vi "Test Executive.vi"(11 "Module Config":T30={"Name"="Test Executive", "Parent Q"=refnum, "Is Child?"=FALSE, "Index"=0, "Dirs"={"Root"=path "C:/MTE", "Config"=path "C:/MTE/Config", "Logs"=path "C:/MTE/Logs", "Reports"=path "C:/ATE/Reports", "App Data"=path "C:/ProgramData/Test Executive"}, "Simulate"=FALSE, "SimCtrl"=refnum}) -> ()   [LabVIEW 2018] (continued)
            n1825 = Delete From Array(array=w3877, index=0) -> (deleted portion=w3874:string, array with subset deleted=w3876:string[])  [unwired: 1 in]
            n1826 = local read "StaCnct"() -> (w3871:bool)
            n1827 = case shown="True" w3871 {
              tunnel: w3876 -> [_ w3915]
              tunnel: w3875 -> [w3890 w3911]
              tunnel: w3874 -> [_ w3896]
              tunnel: w3873 -> [w3887 w3907]
              tunnel: [w3889 w3905] -> w3872
              tunnel: w3870 -> [_ w3898]
              frame False {
                n1828 = call "TestExec.Config, Get Station SW Module Info.vi"() -> ("Sta Exe Path"=w3882:path)  [unwired: 8 in, 3 out]
                n1829 = Strip Path(path=w3882) -> (name=w3881:string)  [unwired: 1 out]
                n1830 = Format Into String(format string="Cannot connect to the '%s'Test Station Applicaiton.\nMake sure it is correctly installed and is running." ("source"), w3881) -> (resulting string=w3883:string)  [unwired: 2 in, 1 out]
                n1831 = call <vilib>:"Q.Enqueue Seq.vi"("Seq Task Name"="Test Running", "Q In"=w3887) -> ()  [unwired: 8 in, 2 out]
                n1832 = Bundle By Name(cluster=errorcluster {"status"=TRUE, "code"=-5100, "source"=""} ("error constant"), "source"=w3883) -> (w3884:errorcluster)
                n1833 = Bundle By Name(cluster=w3890, "ResultError"=w3884) -> (w3889:T73)
              }
              frame True {
                # "Make timeout 10% longer."
                # "Send command to station"
                n1834 = Unbundle By Name(w3911) -> ("TimeOut(s)"=w3917:dbl, "StaApp"=w3912:string)
                n1835 = Multiply(x=1.1, y=w3917) -> (x*y=w3893:dbl)
                n1836 = To Variant(anything=w3915) -> (Variant=w3914:variant)
                n1837 = local read "Abort Flag"() -> (w3892:bool)
                n1838 = Max & Min(x=1.0, y=w3893) -> (min(x,y)=w3894:dbl)  [unwired: 1 out]
                n1839 = call <vilib>:"Q.Enqueue Function.vi"("RetSubCmd"="StaCmd_RTN", "Q Name"=w3912, "Data1"=w3914, "Task Name"=w3896, "Q In"=w3907) -> ("error out"=w3908:errorcluster, "SeqNum"=w3897:i32)  [unwired: 4 in, 1 out]
                n1840 = Select(t=w3894, s=w3892, f=w3893) -> (s? t:f=w3891:dbl)
                n1841 = To Variant(anything=w3896) -> (Variant=w3909:variant)
                n1842 = call <vilib>:"Scheduler.AddTask.vi"("Data1"=w3909, "Interval(s)"=w3891, "Error In"=w3908, "Task Name"="StaCmd_TIMEOUT", "Sched Name"=w3896, "Q In"=w3907) -> ("Error Out"=w3906:errorcluster)  [unwired: 4 in, 1 out]
                n1843 = Bundle By Name(cluster=w3911, "Funct.Seq"=w3897, "Funct.Name"=w3896, "ResultError"=w3906) -> (w3905:T73)
                n1844 = Format Into String(format string="Funct Init: Name \"%s\", Seq %d, TimeOut %#f.", w3896, w3897, w3891) -> (resulting string=w3904:string)  [unwired: 2 in, 1 out]
                n1845 = Unbundle By Name(w3898) -> ("Log"=w3903:refnum<class "Event Notification.lvclass">)
                n1846 = call <vilib>:"Event Notification.Status Message.vi"("Display"=FALSE, "Log"=TRUE, "Level"=Event_Log.Log_Level."Debug0", "Message"=w3904, "Event Notification in"=w3903) -> ()  [unwired: 7 in]
              }
            }
          }
          frame "StaCmd_RTN" {
            n1847 = local read "Abort Flag"() -> (w3919:bool)
            n1848 = Select(t="Done", s=w3919, f="Validate") -> (s? t:f=w3920:string)
            n1849 = while {
              shift-right: [w3935] -> w3924
              shift-left: w3928 -> [w3940]
              tunnel: w3927 -> [w3939]
              tunnel: w3926 -> [w3938]
              tunnel: w3925 -> [w3937]
              shift-right: [w3936] -> _
              shift-left: w3920 -> [w3929]
              tunnel: w3923 -> [w3933]
              shift-right: [w3932] -> _
              shift-left: _ -> [w3931]
              tunnel: w3922 -> [w3930]
              stop <- w3934 stop-if-true
              n1850 = case shown="\"Check Error\"" w3929 {
                tunnel: w3940 -> [w3955 w3964 w3967 w3985 w4007 w4013]
                tunnel: w3939 -> [_ _ w3970 _ _ _]
                tunnel: w3938 -> [w3961 _ _ _ _ _]
                tunnel: w3937 -> [_ _ _ _ _ _]
                tunnel: [w3956 "Load Vars" "Check Error" "Resume Seq" "Done" _] -> w3936
                tunnel: [w3955 w3964 w3971 w3988 w4006 w4013] -> w3935
                tunnel: [_ _ _ _ _ TRUE] -> w3934
                tunnel: w3933 -> [_ w3962 _ _ w4008 _]
                tunnel: [w3945 w3966 w3968 w3987 w4004 w4011] -> w3932
                tunnel: w3931 -> [_ w3966 w3968 w3987 w4004 w4011]
                tunnel: w3930 -> [w3949 _ _ _ _ _]
                frame "Validate" {
                  # "Ignore"
                  n1851 = Variant To Data(type=T55 {"SeqNum"=0, "Data"=variant, "Error"={"status"=FALSE, "code"=0, "source"=""}} ("Ret"), Variant=w3961) -> (data=w3945:T55)  [unwired: 1 in, 1 out]
                  n1852 = Unbundle By Name(w3955) -> ("Funct.Seq"=w3948:i32)
                  n1853 = Unbundle By Name(w3945) -> ("SeqNum"=w3960:i32)
                  n1854 = Unbundle By Name(w3945) -> ("Error.status"=w3944:bool)
                  n1855 = Equal?(x=w3948, y=w3960) -> (x = y?=w3959:bool)
                  n1856 = Select(t="Error", s=w3944, f="OK") -> (s? t:f=w3941:string)
                  n1857 = Select(t="Kill Timeout", s=w3959, f="Done") -> (s? t:f=w3956:string)
                  n1858 = Format Into String(format string="Funct RTN: Seq %d, Status %s", w3948, w3941) -> (resulting string=w3946:string)  [unwired: 2 in, 1 out]
                  n1859 = Unbundle By Name(w3949) -> ("Log"=w3953:refnum<class "Event Notification.lvclass">)
                  n1860 = call <vilib>:"Event Notification.Status Message.vi"("Display"=FALSE, "Log"=TRUE, "Level"=Event_Log.Log_Level."Debug0", "Message"=w3946, "Event Notification in"=w3953) -> ()  [unwired: 7 in]
                }
                frame "Kill Timeout" {
                  n1861 = Unbundle By Name(w3964) -> ("Funct.Name"=w3963:string)
                  n1862 = call <vilib>:"Scheduler.Delete Task.vi"("Sched Name"=w3963, "Q In"=w3962) -> ()  [unwired: 8 in, 2 out]
                }
                frame "Load Vars" {
                  n1863 = Variant To Data(type=string[][] [], Variant=w3970) -> (data=w3972:string[][], error out=w3973:errorcluster)  [unwired: 1 in]
                  n1864 = case shown="No Error" w3973 {
                    tunnel: w3972 -> [w3976 _]
                    tunnel: w3967 -> [w3981 w3982]
                    tunnel: [w3980 w3982] -> w3971
                    frame No Error {
                      n1865 = local read "Variables"() -> (w3977:string[][])
                      n1866 = Unbundle By Name(w3981) -> ("SeqMgr"=w3979:refnum<class "SeqMgr.lvclass">)
                      n1867 = call "TestExec.Add New 1D Items to 2D List, Overwrite if is existing.vi"("New Items"=w3976, "Item List"=w3977) -> ("Item List Out"=w3975:string[][])  [unwired: 9 in]
                      n1868 = call <vilib>:"SeqMgr.Variables - Add, Replace.vi"("Name, Value"=w3976, "SeqMgr in"=w3979) -> ("SeqMgr out"=w3978:refnum<class "SeqMgr.lvclass">)  [unwired: 8 in, 1 out]
                      n1869 = local write "Variables"(w3975) -> ()
                      n1870 = Bundle By Name(cluster=w3981, "SeqMgr"=w3978) -> (w3980:T73)
                    }
                    frame Error {
                      # "No data\nDo nothing"
                    }
                  }
                }
                frame "Check Error" {
                  n1871 = Unbundle By Name(w3985) -> ("Funct.Name"=w3984:string)
                  n1872 = Unbundle By Name(w3987) -> ("Error"=w3986:errorcluster)
                  n1873 = case shown="Error" w3986 {
                    selector: w3986 -> [_ w4001]
                    tunnel: w3984 -> [_ w3998]
                    tunnel: [_ w4000] -> w3983
                    frame No Error {
                    }
                    frame Error {
                      n1874 = Unbundle By Name(w4001) -> ("source"=w3991:string)
                      n1875 = Match Pattern(string=w3991, regular expression="Details = ") -> (after substring=w3992:string, offset past match=w3995:i32)  [unwired: 1 in, 2 out]
                      n1876 = Concatenate Strings("Action = ", w3998) -> (w3997:string)
                      n1877 = Greater Or Equal To 0?(x=w3995) -> (x >= 0?=w3993:bool)
                      n1878 = Select(t=w3992, s=w3993, f=w3991) -> (s? t:f=w3990:string)
                      n1879 = Concatenate Strings(w3997, ", Details = ", w3990) -> (w4002:string)
                      n1880 = Bundle By Name(cluster=w4001, "source"=w4002) -> (w4000:errorcluster)
                    }
                  }
                  n1881 = Bundle By Name(cluster=w3985, "ResultError"=w3983) -> (w3988:T73)
                }
                frame "Resume Seq" {
                  n1882 = call <vilib>:"Q.Enqueue Seq.vi"("Seq Task Name"="Test Running", "Q In"=w4008) -> ()  [unwired: 8 in, 2 out]
                  n1883 = Bundle By Name(cluster=w4007, "Funct.Seq"=0 ("FunctID"), "Funct.Name"="") -> (w4006:T73)
                }
                frame "Done", Default {
                }
              }
            }
          }
          frame "StaCmd_TIMEOUT" {
            n1884 = Unbundle By Name(w4021) -> ("Funct.Name"=w4014:string, "TimeOut(s)"=w4016:dbl, "Funct.Seq"=w4017:i32)
            n1885 = Empty String/Path?(string/path=w4014) -> (empty?=w4015:bool)
            n1886 = case shown="False" w4015 {
              tunnel: w4021 -> [w4041 w4046]
              tunnel: w4020 -> [w4036 _]
              tunnel: [w4032 w4046] -> w4019
              tunnel: w4018 -> [w4031 _]
              tunnel: w4014 -> [w4029 _]
              tunnel: w4017 -> [w4024 _]
              tunnel: w4016 -> [w4023 _]
              frame False {
                n1887 = local read "Test State"() -> (w4035:enum32{"Idle", "Running", "Completed"})
                n1888 = Equal?(x=w4035, y=enum32{"Idle", "Running", "Completed"}."Running" ("Test State")) -> (x = y?=w4033:bool)
                n1889 = case shown="True" w4033 {
                  tunnel: w4036 -> [_ w4044]
                  frame False {
                  }
                  frame True {
                    n1890 = call <vilib>:"Q.Enqueue Seq.vi"("Seq Task Name"="Test Running", "Q In"=w4044) -> ()  [unwired: 8 in, 2 out]
                  }
                }
                n1891 = Format Into String(format string="Function \"%s\" TIMED OUT.  There was no Response within %f# seconds.", w4029, w4023) -> (resulting string=w4038:string)  [unwired: 2 in, 1 out]
                n1892 = Bundle By Name(cluster=errorcluster {"status"=TRUE, "code"=-5100, "source"=""} ("error constant"), "source"=w4038) -> (w4037:errorcluster)
                n1893 = Bundle By Name(cluster=w4041, "Funct.Seq"=0, "Funct.Name"="", "ResultError"=w4037) -> (w4032:T73)
                n1894 = Format Into String(format string="Funct Timeout: Name \"%s\", Seq %d, Time %#f.", w4029, w4024, w4023) -> (resulting string=w4022:string)  [unwired: 2 in, 1 out]
                n1895 = Unbundle By Name(w4031) -> ("Log"=w4030:refnum<class "Event Notification.lvclass">)
                n1896 = call <vilib>:"Event Notification.Status Message.vi"("Display"=FALSE, "Log"=TRUE, "Level"=Event_Log.Log_Level."Verbose", "Message"=w4022, "Event Notification in"=w4030) -> ()  [unwired: 7 in]
              }
              frame True {
                # "Do nothing\nTime out was invalid"
              }
            }
          }
          frame "StaTest End" {
            n1897 = Unbundle By Name(w4049) -> ("StaApp"=w4052:string)
            n1898 = call <vilib>:"Q.Enqueue Task.vi"("Q Name"=w4052, "Task Name"="Test End") -> ()  [unwired: 8 in, 2 out]
            n1899 = call <vilib>:"Q.Enqueue Task.vi"("Q Name"="Wiggler", "Task Name"="Test End") -> ()  [unwired: 8 in, 2 out]
          }
          frame "StaTest Start" {
            n1900 = Unbundle By Name(w4065) -> ("StaApp"=w4055:string, "Data Dirs.Station Data"=w4053:T23[], "RptHdr.Test Sequence.Name"=w4060:string, "RptHdr.Test Run.Start Time"=w4059:timestamp, "RptUUT.UUTInfo.SN"=w4058:string)
            n1901 = Bundle By Name(cluster=T56 {"Test Name"="", "Start Time"=timestamp(0 s since 1904-01-01), "UUT SN"=""} ("Test Start Info"), "Test Name"=w4060, "Start Time"=w4059, "UUT SN"=w4058) -> (w4061:T56)
            n1902 = call <vilib>:"Q.Enqueue Task.vi"("Q Name"=w4055, "Task Name"="Test Reset") -> ()  [unwired: 8 in, 2 out]
            n1903 = To Variant(anything=w4061) -> (Variant=w4063:variant)
            n1904 = To Variant(anything=w4053) -> (Variant=w4054:variant)
            n1905 = call <vilib>:"Q.Enqueue Task.vi"("Data1"=w4054, "Q Name"=w4055, "Task Name"="Test Data Dirs") -> ()  [unwired: 7 in, 2 out]
            n1906 = call <vilib>:"Q.Enqueue Task.vi"("Data1"=w4063, "Q Name"=w4055, "Task Name"="Test Start") -> ()  [unwired: 7 in, 2 out]
          }
          frame "Station Module - Dock" {
            n1907 = call "TestExec.Config, Get Station Module Dock State.vi"() -> ("Dock?"=w4067:bool)  [unwired: 11 in]
            n1908 = case shown="True" w4067 {
              tunnel: w4069 -> [_ w4081]
              tunnel: [_ w4078] -> w4068
              frame False {
                w4073 = refnum<vi> refnum  # TabControl
                n1909 = control-ref of="Funct Tab"() -> (w4075:refnum<vi>)
                n1910 = To More Generic Class(target class=w4073, reference=w4075) -> (generic class reference=w4074:refnum<vi>)
                n1911 = call <vilib>:"CtrlUtil.ShowHide Tab Page.vi"("Show"=FALSE, "Tab Name"="Station Control", "Tab Control"=w4074) -> ()  [unwired: 2 in]
              }
              frame True {
                n1912 = Unbundle By Name(w4081) -> ("App.Child Modules"=w4080:cluster{"VI Ref":refnum<vi>, "Name":string}[])
                n1913 = Index Array(array=w4080) -> (element=w4079:cluster{"VI Ref":refnum<vi>, "Name":string})  [unwired: 1 in]
                n1914 = Unbundle By Name(w4079) -> ("VI Ref"=w4077:refnum<vi>)
                n1915 = Not A Number/Path/Refnum?(number/path/refnum=w4077) -> (NaN/Path/Refnum?=w4076:bool)
                n1916 = case shown="True" w4076 {
                  tunnel: [_ w4083] -> w4078
                  tunnel: w4077 -> [_ w4082]
                  frame False {
                  }
                  frame True {
                    n1917 = invoke on="Sta Ctrl Panel" class="SubPnl" method="Insert VI"("VI Ref"=w4082) -> (error out=w4083:errorcluster)  [unwired: 3 in, 3 out]
                  }
                }
              }
            }
          }
          frame "Station Module - Show" {
            n1918 = Unbundle By Name(w4085) -> ("StaApp"=w4084:string)
            n1919 = call <vilib>:"Module.Window, Q Task.vi"("Q Name"=w4084, "Show"=TRUE, "Action"=Window.Task,_Action."Show Panel(Bool)") -> ()  [unwired: 7 in, 2 out]
          }
          frame "Status" {
            n1920 = Variant To Data(type="", Variant=w4094) -> (data=w4091:string)  [unwired: 1 in, 1 out]
            n1921 = Unbundle By Name(w4089) -> ("Log"=w4096:refnum<class "Event Notification.lvclass">)
            n1922 = Not Equal?(x=w4091, y="Cleared Errors") -> (x != y?=w4090:bool)
            n1923 = case shown="True" w4090 {
              tunnel: w4096 -> [_ w4098]
              tunnel: w4091 -> [_ w4097]
              frame False {
              }
              frame True {
                n1924 = call <vilib>:"Event Notification.Status Message.vi"("Message"=w4097, "Event Notification in"=w4098) -> ()  [unwired: 10 in]
              }
            }
          }
          frame "Subscribe" {
            n1925 = Variant To Data(type=T58 {"Name"="", "Msg"={"Cmd"="", "Sub"="", "Data1"=variant, "Data2"=variant}} ("Subscription"), Variant=w4108) -> (data=w4102:T58)  [unwired: 1 in, 1 out]
            n1926 = Unbundle By Name(w4101) -> ("Subscr"=w4103:T58[])
            n1927 = for {
              tunnel: w4103 -> [w4118] mode=indexing
              tunnel: [w4117] -> w4106 mode=indexing
              n1928 = Unbundle By Name(w4118) -> ("Name"=w4117:string)
            }
            n1929 = Unbundle By Name(w4102) -> ("Name"=w4105:string)
            n1930 = Search 1D Array(1D array=w4106, element=w4105) -> (index of element=w4104:i32)  [unwired: 1 in]
            n1931 = case shown="0, Default" w4104 {
              selector: w4104 -> [w4111 _]
              tunnel: w4103 -> [w4113 w4116]
              tunnel: w4102 -> [w4110 w4115]
              tunnel: [w4112 w4114] -> w4099
              frame 0, Default {
                n1932 = Replace Array Subset(array=w4113, new element=w4110, index=w4111) -> (w4112:T58[])
              }
              frame -1 {
                n1933 = Build Array (concatenate)(w4116, w4115) -> (w4114:T58[])
              }
            }
            n1934 = Bundle By Name(cluster=w4101, "Subscr"=w4099) -> (w4100:T73)
          }
          frame "TCP-IP" {
            # "Connect and disconnect events will send a boolean connect status"
            n1935 = Variant To Data(type=FALSE, Variant=w4130) -> (data=w4127:bool, error out=w4128:errorcluster)  [unwired: 1 in]
            n1936 = case shown="No Error" w4128 {
              tunnel: w4127 -> [w4131 _]
              tunnel: [w4131 _] -> w4119
              frame No Error {
              }
              frame Error {
              }
            }
            n1937 = local write "StaCnct"(w4119) -> ()
            n1938 = Unbundle By Name(w4123) -> ("Log"=w4125:refnum<class "Event Notification.lvclass">)
            n1939 = Select(t="TCP-IP Connected", s=w4119, f="TCP-IP Disconnected") -> (s? t:f=w4120:string)
            n1940 = call <vilib>:"Event Notification.Status Message.vi"("Level"=Event_Log.Log_Level."Verbose", "Message"=w4120, "Event Notification in"=w4125) -> ()  [unwired: 9 in]
          }
          frame "Test Metrics - Add" {
            w4158 = T16 {"TimeStamp"=timestamp(0 s since 1904-01-01), "Dur(s)"=0.0, "Time"="", "Mode "="", "Test "="", "SN"="", "State"=enum."None", "Code"=0, "Description"=""}  # Test Record
            n1941 = Unbundle By Name(w4155) -> ("RptHdr.Test Run.Mode"=w4142:string, "RptHdr.Test Sequence.Name"=w4154:string, "RptUUT.UUTInfo.SN"=w4153:string)
            n1942 = local read "Result Status"() -> (w4156:T2)
            n1943 = local read "Start Time"() -> (w4141:timestamp)
            n1944 = Unbundle By Name(w4156) -> ("State"=w4134:T1, "Code"=w4133:i32, "Description"=w4132:string)
            n1945 = call <vilib>:"Q.Enqueue Task.vi"("Task Name"="Test Metrics - Update Summary", "Q In"=w4136) -> ("Q Out"=w4135:refnum<queue>)  [unwired: 8 in, 1 out]
            n1946 = Format Date/Time String(time format string (%c)="%m/%d/%Y %H:%M:%S", seconds (now)=w4141) -> (date/time string=w4139:string)  [unwired: 1 in]
            n1947 = Unbundle By Name(w4152) -> ("Cfg.Dirs.Logs"=w4145:path)
            n1948 = local read "Duration(s)"() -> (w4143:dbl)
            n1949 = Bundle By Name(cluster=w4158, "TimeStamp"=w4141, "Time"=w4139, "Dur(s)"=w4143, "Mode"=w4142, "Test"=w4154, "SN"=w4153, "State"=w4134, "Code"=w4133, "Description"=w4132) -> (w4157:T16)
            n1950 = call "TestExec.Test Metric Add_Get.vi"("Log Dir"=w4145, "Test Record"=w4157, "Action"=TestExec.Test_Metric_Action_Selector."Append", "Test Result Metrics"="Test Result Metrics") -> ("Test History"=w4151:T15, "Test Result Metrics Out"=w4159:T3)  [unwired: 6 in]
            n1951 = case shown="\"ABORT\"" w4134 {
              tunnel: w4135 -> [_ w4165 _]
              tunnel: w4133 -> [_ w4161 _]
              tunnel: w4132 -> [_ w4160 _]
              frame "None", Default {
              }
              frame "ERROR" {
                n1952 = Bundle By Name(cluster=errorcluster {"status"=TRUE, "code"=0, "source"=""} ("error constant"), "status"=TRUE, "code"=w4161, "source"=w4160) -> (w4162:errorcluster)
                n1953 = call "TestExec.Health, Set Error.vi"("Error"=w4162, "Q In"=w4165) -> ()  [unwired: 9 in, 1 out]
              }
              frame "ABORT" {
                # "Do Nothing"
              }
            }
            n1954 = local write "Test Result Metrics"(w4159) -> ()
            n1955 = call "TestExec.Test Metric Pareto.vi"("Test History"=w4151) -> ("Counts"=w4149:i32[], "Codes"=w4150:i32[])  [unwired: 9 in]
            n1956 = local write "Test History"(w4151) -> ()
            n1957 = Build Array(w4150, w4149) -> (w4148:i32[][])
            n1958 = Transpose 2D Array(2D array=w4148) -> (transposed array=→"Pareto":i32[][])
            n1959 = property on="Test History" class="Arr (strict)"("Index Values"=u32[] [0]) -> ()  [unwired: 2 in, 2 out]
          }
          frame "Test Metrics - Load" {
            n1960 = Unbundle By Name(w4177) -> ("Cfg.Dirs.Logs"=w4176:path)
            n1961 = local read "Test Result Metrics"() -> (w4170:T3)
            n1962 = call <vilib>:"Q.Enqueue Task.vi"("Top of Q"=TRUE, "Task Name"="Test Metrics - Update Summary", "Q In"=w4167) -> ()  [unwired: 7 in, 2 out]
            n1963 = call "TestExec.Test Metric Add_Get.vi"("Log Dir"=w4176, "Action"=TestExec.Test_Metric_Action_Selector."Load", "Test Result Metrics"=w4170) -> ("Test History"=w4171:T15, "Test Result Metrics Out"=w4178:T3)  [unwired: 7 in]
            n1964 = local write "Test Result Metrics"(w4178) -> ()
            n1965 = call "TestExec.Test Metric Pareto.vi"("Test History"=w4171) -> ("Counts"=w4174:i32[], "Codes"=w4175:i32[])  [unwired: 9 in]
            n1966 = local write "Test History"(w4171) -> ()
            n1967 = Build Array(w4175, w4174) -> (w4173:i32[][])
            n1968 = local write "Pareto"(w4173) -> ()
            n1969 = property on="Test History" class="Arr (strict)"("Index Values"=u32[] [0]) -> ()  [unwired: 2 in, 2 out]
          }
          frame "Test Metrics - Reset" {
            n1970 = Unbundle By Name(w4186) -> ("Cfg.Dirs.Logs"=w4185:path)
            n1971 = local read "Test Result Metrics"() -> (w4188:T3)
            n1972 = call <vilib>:"Q.Enqueue Task.vi"("Task Name"="Test Metrics - Update Summary", "Q In"=w4180) -> ()  [unwired: 8 in, 2 out]
            n1973 = call "TestExec.Test Metric Add_Get.vi"("Log Dir"=w4185, "Action"=TestExec.Test_Metric_Action_Selector."Reset", "Test Result Metrics"=w4188) -> ("Test History"=w4190:T15, "Test Result Metrics Out"=w4189:T3)  [unwired: 7 in]
            n1974 = local write "Test Result Metrics"(w4189) -> ()
            n1975 = local write "Test History"(w4190) -> ()
            n1976 = local write "Pareto"(i32[][] [] ("Pareto")) -> ()
            n1977 = property on="Test History" class="Arr (strict)"("Index Values"=u32[] [0]) -> ()  [unwired: 2 in, 2 out]
          }
          frame "Test Metrics - Update" {
            n1978 = local read "Test Result Metrics"() -> (w4194:T3)
            n1979 = Unbundle By Name(w4201) -> ("Cfg.Dirs.Logs"=w4200:path)
            n1980 = call <vilib>:"Q.Enqueue Task.vi"("Task Name"="Test Metrics - Update Summary", "Q In"=w4191) -> ()  [unwired: 8 in, 2 out]
            n1981 = call "TestExec.Test Metric Add_Get.vi"("Log Dir"=w4200, "Action"=TestExec.Test_Metric_Action_Selector."Get Metrics", "Test Result Metrics"=w4194) -> ("Test History"=w4197:T15, "Test Result Metrics Out"=w4202:T3)  [unwired: 7 in]
            "Test History" <- w4197
            n1982 = local write "Test Result Metrics"(w4202) -> ()
            n1983 = call "TestExec.Test Metric Pareto.vi"("Test History"=w4197) -> ("Counts"=w4198:i32[], "Codes"=w4199:i32[])  [unwired: 9 in]
            n1984 = Build Array(w4199, w4198) -> (w4196:i32[][])
            n1985 = local write "Pareto"(w4196) -> ()
            n1986 = property on="Test History" class="Arr (strict)"("Index Values"=u32[] [0]) -> ()  [unwired: 2 in, 2 out]
          }
          frame "Test Metrics - Update Summary" {
            n1987 = local read "Test Result Metrics"() -> (w4226:T3)
            n1988 = Unbundle By Name(w4226) -> ("Yield%"=w4224:dbl, "Pass Cnt"=→"Pass Cnt":i32, "Error Cnt"=w4210:i32, "Fail Cnt"=w4209:i32, "Abort Cnt"=w4205:i32)
            "Fail Cnt" <- w4209
            "Yield%" <- w4224
            "Error Cnt" <- w4210
            "Abort Cnt" <- w4205
            n1989 = Less?(x=w4224, y=100.0) -> (x < y?=w4212:bool)
            n1990 = Greater Than 0?(x=w4205) -> (x > 0?=w4208:bool)
            n1991 = Greater Than 0?(x=w4210) -> (x > 0?=w4213:bool)
            n1992 = Greater Than 0?(x=w4209) -> (x > 0?=w4214:bool)
            n1993 = Select(t=u32 16318208, s=w4212, f=u32 6618880) -> (s? t:f=w4221:u32)
            n1994 = Select(t=u32 16711680, s=w4213, f=u32 16448250) -> (s? t:f=w4215:u32)
            n1995 = Select(t=u32 16756242, s=w4208, f=u32 16448250) -> (s? t:f=w4204:u32)
            n1996 = Select(t=u32 16711680, s=w4214, f=u32 16448250) -> (s? t:f=w4216:u32)
            n1997 = property on="Yield%" class="DigNum (strict)"("NumText.BGColor"=w4221) -> ()  [unwired: 2 in, 2 out]
            n1998 = property on="Error Cnt" class="DigNum (strict)"("NumText.BGColor"=w4215) -> ()  [unwired: 2 in, 2 out]
            n1999 = property on="Abort Cnt" class="DigNum (strict)"("NumText.BGColor"=w4204) -> ()  [unwired: 2 in, 2 out]
            n2000 = property on="Fail Cnt" class="DigNum (strict)"("NumText.BGColor"=w4216) -> ()  [unwired: 2 in, 2 out]
          }
          frame "Update Result Table" {
            n2001 = Unbundle By Name(w4235) -> ("Data.FileObjs"=w4230:T29[], "Data.Meas"=w4229:T38[])
            "File Data Objs" <- w4230
            n2002 = call <vilib>:"Q.Enqueue Task.vi"("Top of Q"=TRUE, "Task Name"="Sta Test Status", "Q In"=w4236) -> ()  [unwired: 7 in, 2 out]
            n2003 = call "Result.Attributes plus Numeric into Results Table.vi"("Meas"=w4229, "File Data Objs"=w4230, "Show Only Failures"="Show Only Failures", "Filter"="Filter") -> ("Results Table"=w4231:T7[])  [unwired: 7 in]
            "Results Table" <- w4231
            n2004 = case shown="True" "Auto Scroll" {
              tunnel: w4231 -> [_ w4249]
              frame False {
              }
              frame True {
                w4242 = 14  # Table Rows
                # "Auto Scroll"
                # "Set to num of visible rows"
                n2005 = Array Size(array=w4249) -> (size(s)=w4243:i32)
                n2006 = Decrement(x=w4242) -> (x-1=w4241:i32)
                n2007 = Subtract(x=w4243, y=w4241) -> (x-y=w4245:i32)
                n2008 = Greater Or Equal To 0?(x=w4245) -> (x >= 0?=w4244:bool)
                n2009 = Select(t=w4245, s=w4244, f=0) -> (s? t:f=w4247:i32)
                n2010 = Build Array(w4247) -> (w4248:i32[])
                n2011 = To Unsigned Long Integer(number=w4248) -> (unsigned 32bit integer=w4240:u32[])
                n2012 = property on="Results Table" class="Arr (strict)"("Index Values"=w4240) -> ()  [unwired: 2 in, 2 out]
              }
            }
          }
          frame "UUT - Dir" {
            n2013 = Variant To Data(type=path "", Variant=w4260) -> (data=w4255:path, error out=w4258:errorcluster)  [unwired: 1 in]
            n2014 = Bundle By Name(cluster=w4261, "UUT Dir"=w4255) -> (w4257:T73)
            n2015 = Format Into String(format string="UUT - Dir, %s", w4255) -> (resulting string=w4250:string)  [unwired: 2 in, 1 out]
            n2016 = Unbundle By Name(w4251) -> ("Log"=w4254:refnum<class "Event Notification.lvclass">)
            n2017 = call <vilib>:"Event Notification.Status Message.vi"("Log"=TRUE, "Level"=Event_Log.Log_Level."Verbose", "Message"=w4250, "Event Notification in"=w4254) -> ()  [unwired: 8 in]
          }
          frame "UUT - Properties" {
            # "If name exists, over write.\nElse append."
            # "UUT - Properties(2D array of Str: Name, Value)"
            n2018 = Variant To Data(type=string[][] [], Variant=w4271) -> (data=w4262:string[][])  [unwired: 1 in, 1 out]
            n2019 = Unbundle By Name(w4268) -> ("RptUUT.UUTInfo.Properties.Property"=w4265:cluster{"Name":string, "Value":string}[])
            n2020 = for {
              tunnel: w4265 -> [w4274] mode=indexing
              tunnel: [w4273] -> w4267 mode=indexing
              n2021 = Unbundle By Name(w4274) -> ("Name"=w4273:string)
            }
            n2022 = local read "UUT Properties"() -> (w4264:string[][])
            n2023 = for {
              tunnel: w4262 -> [w4283] mode=indexing
              shift-right: [w4281] -> w4266
              shift-left: w4265 -> [w4282]
              tunnel: w4267 -> [w4276]
              n2024 = Index Array(array=w4283) -> (element #1=w4275:string, element #2=w4279:string)  [unwired: 2 in]
              n2025 = Bundle By Name(cluster=cluster{"Name":string, "Value":string} {"Name"="", "Value"=""} ("Setup"), "Name"=w4275, "Value"=w4279) -> (w4278:cluster{"Name":string, "Value":string})
              n2026 = Search 1D Array(1D array=w4276, element=w4275) -> (index of element=w4277:i32)  [unwired: 1 in]
              n2027 = case shown="0, Default" w4277 {
                selector: w4277 -> [w4284 _]
                tunnel: w4282 -> [w4287 w4290]
                tunnel: [w4286 w4289] -> w4281
                tunnel: w4278 -> [w4285 w4288]
                frame 0, Default {
                  n2028 = Replace Array Subset(array=w4287, new element=w4285, index=w4284) -> (w4286:cluster{"Name":string, "Value":string}[])
                }
                frame -1 {
                  n2029 = Build Array (concatenate)(w4290, w4288) -> (w4289:cluster{"Name":string, "Value":string}[])
                }
              }
            }
            n2030 = call "TestExec.Add New 1D Items to 2D List, Overwrite if is existing.vi"("New Items"=w4262, "Item List"=w4264) -> ("Item List Out"=→"UUT Properties":string[][])  [unwired: 9 in]
            n2031 = Bundle By Name(cluster=w4268, "RptUUT.UUTInfo.Properties.Property"=w4266) -> (w4269:T73)
          }
          frame "Warning" {
            n2032 = Variant To Data(type=w4292, Variant=w4293) -> (data=w4291:errorcluster)  [unwired: 1 in, 1 out]
            n2033 = call "TestExec.Health Status, Set Error_Warning.vi"("error in"=w4291, "Health State Cmd"=TestExec.Health_State_Command."Set Warning", "Q In"=w4294) -> ()  [unwired: 8 in, 1 out]
          }
          frame Default {
            n2034 = Match Pattern(string=w4301, regular expression="^Cmd_") -> (after substring=w4299:string, offset past match=w4300:i32)  [unwired: 1 in, 2 out]
            n2035 = case shown="-1" w4300 {
              tunnel: w4307 -> [_ w4318]
              tunnel: w4306 -> [_ w4317]
              tunnel: w4305 -> [_ w4316]
              tunnel: w4304 -> [_ w4315]
              tunnel: w4301 -> [_ w4314]
              tunnel: w4299 -> [w4312 _]
              tunnel: [w4308 w4313] -> w4298
              frame 0, Default {
                n2036 = Format Into String(format string="Invalid test script command: \"%s\".", w4312) -> (resulting string=w4309:string)  [unwired: 2 in, 1 out]
                n2037 = Bundle By Name(cluster=errorcluster {"status"=TRUE, "code"=-5500, "source"=""} ("error constant"), "source"=w4309) -> (w4308:errorcluster)
              }
              frame -1 {
                n2038 = call <vilib>:"Module.Default Tasks.vi"("Sys"=w4315, "error in"=w4316, "Data2"=w4317, "Data1"=w4318, "Sub"=w4314) -> ("error out"=w4313:errorcluster)  [unwired: 5 in, 1 out]
              }
            }
          }
        }
      }
      frame "Remote" {
        n2039 = case shown="\"True\"" w4319 {
          frame "False", Default {
          }
          frame "True" {
          }
        }
      }
      frame "Seq" {
        n2040 = case shown="\"Test Running\"" w4325 {
          tunnel: w4329 -> [w4331 w4351 w4360 w4531 w4604 w4690 w4746 w4872 w4892 w4946 w5027]
          tunnel: [w4331 w4351 w4359 w4531 w4604 w4690 w4746 w4872 w4892 w4946 w5027] -> w4328
          tunnel: w4327 -> [w4330 w4344 w4352 w4534 w4603 w4689 w4747 w4863 w4879 w4915 w5007]
          tunnel: [w4330 w4343 w4358 w4533 w4644 w4730 w4743 w4863 w4882 w4964 w5046] -> w4326
          tunnel: w4324 -> [_ _ w4353 w4536 w4651 w4695 w4751 _ w4880 w4934 w5034]
          tunnel: w4323 -> [_ _ w4357 w4538 _ _ _ _ _ _ _]
          tunnel: w4322 -> [_ _ w4354 _ _ _ _ _ _ _ _]
          frame Default {
          }
          frame "Init Controls" {
            w4348 = T84 {"Running"=refnum, "StartTime"=refnum, "EndTime"=refnum, "ProgressBar"=refnum, "Duration(s)"=refnum, "Test Ctrl Tab"=refnum, "Failing Status"=refnum}  # ProgressCtrls
            w4347 = T85 {"State"=refnum, "Code"=refnum, "Desc"=refnum, "StateColors"=[13816530, 11009952, 16758968, 6618880, 16711680, 16711680, 16711680]}  # ResultCtrls
            n2041 = control-ref of="Duration(s)"() -> (w4336:refnum<vi>)
            n2042 = control-ref of="End Time"() -> (w4334:refnum<vi>)
            n2043 = control-ref of="Progress"() -> (w4338:refnum<vi>)
            n2044 = control-ref of="Start Time"() -> (w4335:refnum<vi>)
            n2045 = control-ref of="Test Running"() -> (w4337:refnum<vi>)
            n2046 = control-ref of="Code"() -> (w4340:refnum<vi>)
            n2047 = control-ref of="State"() -> (w4332:refnum<vi>)
            n2048 = control-ref of="Description"() -> (w4341:refnum<vi>)
            n2049 = control-ref of="Failing Status"() -> (w4339:refnum<vi>)
            n2050 = control-ref of="Test Ctrl Tab"() -> (w4342:refnum<vi>)
            n2051 = Bundle By Name(cluster=w4348, "Running"=w4337, "StartTime"=w4335, "EndTime"=w4334, "ProgressBar"=w4338, "Duration(s)"=w4336, "Test Ctrl Tab"=w4342, "Failing Status"=w4339) -> (w4346:T84)
            n2052 = Unbundle By Name(w4344) -> ("SeqMgr"=w4350:refnum<class "SeqMgr.lvclass">)
            n2053 = Bundle By Name(cluster=w4347, "State"=w4332, "Code"=w4340, "Desc"=w4341, "StateColors"=u32[] [13816530, 15925128, 16758968, 6618880, 16711680, 16711680, 16711680]) -> (w4345:T85)
            n2054 = call <vilib>:"SeqMgr.Initialize Seq, Init Progress Controls.vi"("ResultCtrls"=w4345, "ProgressCtrls"=w4346, "SeqMgr in"=w4350) -> ("SeqMgr out"=w4349:refnum<class "SeqMgr.lvclass">)  [unwired: 7 in, 1 out]
            n2055 = invoke on="Duration(HH:MM:SS)" class="Str" method="Reinit To Default"() -> ()  [unwired: 3 in, 3 out]
            n2056 = Bundle By Name(cluster=w4344, "SeqMgr"=w4349) -> (w4343:T73)
          }
          frame "Test Idle" {
            n2057 = Variant To Data(type="", Variant=w4357) -> (data=w4355:string)  [unwired: 1 in, 1 out]
            n2058 = case shown="\"Init\", Default" w4355 {
              tunnel: w4360 -> [w4398 w4448 w4483 w4530]
              tunnel: [w4398 w4448 w4483 w4530] -> w4359
              tunnel: w4352 -> [w4371 w4441 w4474 w4529]
              tunnel: [w4397 w4446 w4482 w4529] -> w4358
              tunnel: w4354 -> [_ _ _ _]
              tunnel: w4353 -> [w4363 w4444 w4480 _]
              frame "Init", Default {
                w4381 = T36."Enabled" ("Disabled")
                n2059 = Unbundle By Name(w4371) -> ("PreTestCk.NoSN"=w4368:bool, "Opts.NotValSN"=w4365:bool)
                n2060 = local read "Operator"() -> (w4391:string)
                n2061 = call <vilib>:"Q.Enqueue Task.vi"("Task Name"="Maint - Scheduler" ("Pretest Check.Oper.Desc"), "Q In"=w4363) -> ("Q Out"=w4362:refnum<queue>)  [unwired: 8 in, 1 out]
                n2062 = Unbundle By Name(w4371) -> ("Repeat(s)"=w4389:dbl)
                n2063 = Unbundle By Name(w4371) -> ("Opts.NotValOper"=w4380:bool)
                n2064 = Empty String/Path?(string/path=w4391) -> (empty?=w4396:bool)
                n2065 = property on="Operator" class="Str"("DisabledEnum"=w4381, "Text.BGColor"=u32 16448250) -> ()  [unwired: 2 in, 2 out]
                n2066 = property on="SN" class="Str"("DisabledEnum"=w4381, "Text.BGColor"=u32 16383928) -> ()  [unwired: 2 in, 2 out]
                n2067 = Or(x=w4368, y=w4365) -> (x .or. y?=w4367:bool)
                n2068 = case shown="True" w4367 {
                  tunnel: w4371 -> [w4401 _]
                  tunnel: [w4404 TRUE] -> w4370
                  tunnel: [w4403 _] -> w4369
                  tunnel: [w4399 _] -> _
                  frame False {
                    n2069 = Unbundle By Name(w4401) -> ("Opts.SNRouteCk"=w4405:bool)
                    n2070 = Unbundle By Name(w4401) -> ("Lists.UUTRoutes"=w4402:string[])
                    n2071 = local read "SN"() -> (w4406:string)
                    n2072 = control-ref of="SN"() -> (w4400:refnum<vi>)
                    n2073 = call "TestExec.SN Valid and Route Check.vi"("Process Steps"=w4402, "SN Indicator"=w4400, "SN"=w4406, "Route Check"=w4405) -> ("Message"=w4403:string, "Status"=w4404:bool, "error IO"=w4399:errorcluster)  [unwired: 4 in, 1 out]
                  }
                  frame True {
                  }
                }
                n2074 = Not(x=w4396) -> (.not. x?=w4383:bool)
                n2075 = Greater Or Equal To 0?(x=w4389) -> (x >= 0?=w4384:bool)
                n2076 = call <vilib>:"Q.Enqueue Task.vi"("Task Name"="Sta Notify" ("Pretest Check.Oper.Desc"), "Q In"=w4362) -> ("Q Out"=w4378:refnum<queue>)  [unwired: 8 in, 1 out]
                n2077 = Or(x=w4380, y=w4383) -> (x .or. y?=w4390:bool)
                n2078 = Or(x=w4390, y=w4370) -> (x .or. y?=w4387:bool)
                n2079 = local read "Test Status Tab"() -> (w4374:T6)
                n2080 = And(x=w4390, y=w4370) -> (x .and. y?=w4385:bool)
                n2081 = property on="SN" class="Str"("Key Focus"=TRUE) -> ()  [unwired: 2 in, 2 out]
                n2082 = Or(x=w4384, y=w4387) -> (x .or. y?=w4388:bool)
                n2083 = Or(x=w4384, y=w4385) -> (x .or. y?=w4386:bool)
                n2084 = To Unsigned Long Integer(number=w4374) -> (unsigned 32bit integer=w4375:u32)
                n2085 = case shown="True" w4388 {
                  tunnel: ["Enter Operator and UUT SN to begin a test." w4416] -> w4393
                  tunnel: [T36."Disabled and Grayed Out" ("Disabled") w4415] -> w4392
                  tunnel: w4386 -> [_ w4414]
                  tunnel: w4378 -> [_ w4413]
                  tunnel: w4370 -> [_ w4412]
                  tunnel: w4369 -> [_ w4411]
                  frame False {
                    n2086 = property on="SN" class="Str"("Key Focus"=TRUE) -> ()  [unwired: 2 in, 2 out]
                  }
                  frame True {
                    n2087 = case shown="True" w4414 {
                      tunnel: [w4420 "Click Start to run a test"] -> w4416
                      tunnel: w4413 -> [_ w4430]
                      tunnel: [w4419 T36."Enabled" ("Disabled")] -> w4415
                      tunnel: w4412 -> [w4418 _]
                      tunnel: w4411 -> [w4417 _]
                      frame False {
                        n2088 = case shown="True" w4418 {
                          tunnel: [w4421 "Enter a valid Operator to begin a test."] -> w4420
                          tunnel: [T36."Disabled and Grayed Out" ("Disabled") T36."Disabled and Grayed Out" ("Disabled")] -> w4419
                          tunnel: w4417 -> [w4421 _]
                          frame False {
                            n2089 = property on="SN" class="Str"("Key Focus"=TRUE) -> ()  [unwired: 2 in, 2 out]
                          }
                          frame True {
                            n2090 = property on="Operator" class="Str"("Key Focus"=TRUE) -> ()  [unwired: 2 in, 2 out]
                          }
                        }
                      }
                      frame True {
                        n2091 = property on="Start" class="Bool"("Key Focus"=TRUE) -> ()  [unwired: 2 in, 2 out]
                        n2092 = To Variant(anything="Ready") -> (Variant=w4433:variant)
                        n2093 = call <vilib>:"Q.Enqueue Seq.vi"("Top of Q"=TRUE, "Data1"=w4433, "Seq Task Name"="Test Idle", "Q In"=w4430) -> ()  [unwired: 6 in, 2 out]
                      }
                    }
                  }
                }
                n2094 = In Range and Coerce(upper limit=u32 1, x=w4375, lower limit=u32 0) -> (coerced(x)=w4364:u32)  [unwired: 1 out]
                n2095 = local write "Test Status Tab Sel"(w4364) -> ()
                n2096 = local write "Test Status Tab"(w4364) -> ()
                n2097 = Bundle By Name(cluster=w4371, "PreTestCk.Oper.OK"=w4390, "PreTestCk.Oper.Desc"="" ("Pretest Check.Oper.Desc"), "PreTestCk.SN.OK"=w4370, "PreTestCk.SN.Desc"="" ("Pretest Check.Oper.Desc"), "PreTestCk.SNErr"=FALSE) -> (w4397:T73)
                n2098 = local write "UUT SN Status"(w4393) -> ()
                n2099 = property on="Start" class="Bool"("DisabledEnum"=w4392) -> ()  [unwired: 2 in, 2 out]
              }
              frame "Operator Change" {
                n2100 = Unbundle By Name(w4441) -> ("Opts.NotValOper"=w4438:bool, "PreTestCk.SN.OK"=w4437:bool, "Opts.NotValSN"=w4436:bool)
                n2101 = control-ref of="Operator"() -> (w4447:refnum<vi>)
                n2102 = call "TestExec.Operator Validation Check.vi"("String"=w4447) -> ("Description"=w4443:string, "OK"=w4439:bool)  [unwired: 9 in]
                n2103 = Or(x=w4437, y=w4436) -> (x .or. y?=w4435:bool)
                n2104 = Or(x=w4439, y=w4438) -> (x .or. y?=w4440:bool)
                n2105 = Bundle By Name(cluster=w4441, "PreTestCk.Oper.OK"=w4439, "PreTestCk.Oper.Desc"=w4443) -> (w4446:T73)
                n2106 = case shown="True" w4440 {
                  tunnel: [w4451 w4457] -> w4445
                  tunnel: w4435 -> [_ w4456]
                  tunnel: w4444 -> [_ w4455]
                  tunnel: w4443 -> [w4452 _]
                  tunnel: [T36."Disabled and Grayed Out" ("Disabled") w4454] -> w4442
                  frame False {
                    n2107 = property on="Operator" class="Str"("Key Focus"=TRUE) -> ()  [unwired: 2 in, 2 out]
                    n2108 = Format Into String(format string="The operator entered was invalid: %s\n\nEnter Operator and UUT SN to begin a test.", w4452) -> (resulting string=w4451:string)  [unwired: 2 in, 1 out]
                  }
                  frame True {
                    n2109 = case shown="True" w4456 {
                      tunnel: ["Enter UUT SN to begin a test." "Click Start to run a test"] -> w4457
                      tunnel: w4455 -> [_ w4464]
                      tunnel: [T36."Disabled and Grayed Out" ("Disabled") T36."Enabled" ("Disabled")] -> w4454
                      frame False {
                        n2110 = property on="SN" class="Str"("Key Focus"=TRUE) -> ()  [unwired: 2 in, 2 out]
                      }
                      frame True {
                        n2111 = property on="Start" class="Bool"("Key Focus"=TRUE) -> ()  [unwired: 2 in, 2 out]
                        n2112 = To Variant(anything="Ready") -> (Variant=w4467:variant)
                        n2113 = call <vilib>:"Q.Enqueue Seq.vi"("Top of Q"=TRUE, "Data1"=w4467, "Seq Task Name"="Test Idle", "Q In"=w4464) -> ()  [unwired: 6 in, 2 out]
                      }
                    }
                  }
                }
                n2114 = local write "UUT SN Status"(w4445) -> ()
                n2115 = property on="Start" class="Bool"("DisabledEnum"=w4442) -> ()  [unwired: 2 in, 2 out]
              }
              frame "SN Change" {
                n2116 = Unbundle By Name(w4474) -> ("PreTestCk.NoSN"=w4470:bool, "Opts.NotValSN"=w4469:bool, "Opts.NotValOper"=w4475:bool, "PreTestCk.Oper.OK"=w4478:bool)
                n2117 = Or(x=w4470, y=w4469) -> (x .or. y?=w4471:bool)
                n2118 = case shown="False" w4471 {
                  tunnel: w4474 -> [w4486 _]
                  tunnel: [w4489 TRUE] -> w4472
                  tunnel: [w4488 _] -> w4473
                  tunnel: [w4484 _] -> _
                  frame False {
                    n2119 = Unbundle By Name(w4486) -> ("Lists.UUTRoutes"=w4487:string[])
                    n2120 = Unbundle By Name(w4486) -> ("Opts.SNRouteCk"=w4490:bool)
                    n2121 = local read "SN"() -> (w4491:string)
                    n2122 = control-ref of="SN"() -> (w4485:refnum<vi>)
                    n2123 = call "TestExec.SN Valid and Route Check.vi"("Process Steps"=w4487, "SN Indicator"=w4485, "SN"=w4491, "Route Check"=w4490) -> ("Message"=w4488:string, "Status"=w4489:bool, "error IO"=w4484:errorcluster)  [unwired: 4 in, 1 out]
                  }
                  frame True {
                  }
                }
                n2124 = Or(x=w4475, y=w4478) -> (x .or. y?=w4477:bool)
                n2125 = case shown="True" w4472 {
                  tunnel: [w4495 w4508] -> w4481
                  tunnel: w4477 -> [w4499 w4507]
                  tunnel: w4480 -> [_ w4506]
                  tunnel: w4473 -> [w4503 _]
                  tunnel: [T36."Disabled and Grayed Out" ("Disabled") w4505] -> w4479
                  tunnel: "Start with SN Entry" -> [_ w4504]
                  frame False {
                    n2126 = property on="SN" class="Str"("Key Focus"=TRUE) -> ()  [unwired: 2 in, 2 out]
                    n2127 = Format Into String(format string="The SN entered was rejected: %s", w4503) -> (resulting string=w4501:string)  [unwired: 2 in, 1 out]
                    n2128 = Select(t="Enter UUT SN to begin a test.", s=w4499, f="Enter Operator and UUT SN to begin a test.") -> (s? t:f=w4496:string)
                    n2129 = Concatenate Strings(w4501, "\r\n", w4496) -> (w4495:string)
                  }
                  frame True {
                    n2130 = case shown="True" w4507 {
                      tunnel: ["Enter a valid Operator to begin a test." w4512] -> w4508
                      tunnel: w4506 -> [_ w4515]
                      tunnel: [T36."Disabled and Grayed Out" ("Disabled") w4513] -> w4505
                      tunnel: w4504 -> [_ w4514]
                      frame False {
                        n2131 = property on="Operator" class="Str"("Key Focus"=TRUE) -> ()  [unwired: 2 in, 2 out]
                      }
                      frame True {
                        n2132 = case shown="False" w4514 {
                          tunnel: w4515 -> [w4519 w4525]
                          tunnel: [T36."Enabled" ("Disabled") T36."Disabled and Grayed Out" ("Disabled")] -> w4513
                          tunnel: ["Click Start to run a test" "Auto Starting test"] -> w4512
                          frame False {
                            n2133 = property on="Start" class="Bool"("Key Focus"=TRUE) -> ()  [unwired: 2 in, 2 out]
                            n2134 = To Variant(anything="Ready") -> (Variant=w4522:variant)
                            n2135 = call <vilib>:"Q.Enqueue Seq.vi"("Data1"=w4522, "Seq Task Name"="Test Idle", "Q In"=w4519) -> ()  [unwired: 7 in, 2 out]
                          }
                          frame True {
                            n2136 = call <vilib>:"Q.Enqueue Seq.vi"("Seq Task Name"="Test Start", "Q In"=w4525) -> ()  [unwired: 8 in, 2 out]
                          }
                        }
                      }
                    }
                  }
                }
                n2137 = Bundle By Name(cluster=w4474, "PreTestCk.SN.OK"=w4472, "PreTestCk.SN.Desc"=w4473) -> (w4482:T73)
                n2138 = local write "UUT SN Status"(w4481) -> ()
                n2139 = property on="Start" class="Bool"("DisabledEnum"=w4479) -> ()  [unwired: 2 in, 2 out]
              }
              frame "Ready" {
                n2140 = property on="Start" class="Bool"("Key Focus"=TRUE) -> ()  [unwired: 2 in, 2 out]
                n2141 = property on="Start" class="Bool"("DisabledEnum"=T36."Enabled" ("Disabled")) -> ()  [unwired: 2 in, 2 out]
              }
            }
          }
          frame "Remote Test Start" {
            n2142 = local read "Test State"() -> (w4535:enum32{"Idle", "Running", "Completed"})
            n2143 = Variant To Data(type=T61 {"Sequence"="", "SN"="", "Pos"=""}, Variant=w4538) -> (data=w4532:T61)  [unwired: 1 in, 1 out]
            n2144 = case shown="\"Idle\", \"Completed\"" w4535 {
              tunnel: w4536 -> [w4543 w4561]
              tunnel: w4534 -> [w4553 w4560]
              tunnel: [w4553 w4559] -> w4533
              tunnel: w4532 -> [w4545 w4558]
              tunnel: w4531 -> [w4546 w4555]
              frame "Running", Default {
                # "Do Nothing.\nNot in a state to run a new test"
                n2145 = Unbundle By Name(w4545) -> ("Sequence"=w4539:string, "SN"=w4544:string)
                n2146 = Empty String/Path?(string/path=w4539) -> (empty?=w4552:bool)
                n2147 = Select(t="Default", s=w4552, f=w4539) -> (s? t:f=w4550:string)
                n2148 = Format Into String(format string="Remote Test Launch IGNORED since test state is running.  Request was Seq = %s, SN = %s" ("Message"), w4550, w4544) -> (resulting string=w4540:string)  [unwired: 2 in, 1 out]
                n2149 = Unbundle By Name(w4546) -> ("Log"=w4548:refnum<class "Event Notification.lvclass">)
                n2150 = call <vilib>:"Event Notification.Status Message.vi"("Log"=TRUE, "Message"=w4540, "Event Notification in"=w4548) -> ()  [unwired: 9 in]
                n2151 = Bundle By Name(cluster=errorcluster {"status"=FALSE, "code"=7000, "source"=""} ("Error"), "source"=w4540) -> (w4541:errorcluster)
                n2152 = call "TestExec.Health, Set Warning.vi"("Error"=w4541, "Q In"=w4543) -> ()  [unwired: 9 in, 1 out]
              }
              frame "Idle", "Completed" {
                n2153 = Unbundle By Name(w4558) -> ("Sequence"=w4557:string)
                n2154 = case shown="Default" w4557 {
                  selector: w4557 -> [_ w4563]
                  tunnel: [_ w4565] -> w4556
                  tunnel: ["Default" w4564] -> w4554
                  frame "" {
                    # "No Seq"
                  }
                  frame Default {
                    n2155 = property on="Sequence" class="Ring (strict)"() -> ("Strings []"=w4566:string[])  [unwired: 2 in, 2 out]
                    n2156 = To Lower Case(string=w4563) -> (all lower case string=w4568:string)
                    n2157 = To Lower Case(string=w4566) -> (all lower case string=w4567:string[])
                    n2158 = Search 1D Array(1D array=w4567, element=w4568) -> (index of element=w4569:i32)  [unwired: 1 in]
                    n2159 = case shown="0, Default" w4569 {
                      selector: w4569 -> [_ w4577]
                      tunnel: w4563 -> [w4571 w4576]
                      tunnel: [w4570 _] -> w4565
                      tunnel: [_ w4576] -> w4564
                      frame -1 {
                        w4574 = T74 -6100 items=["No Error"=0, "Abort"=-2, "Misc"=-5000, "Fixture Error"=-5100, "File IO - General"=-5200, "FIle IO - Config Error"=-5201, "Instrument - General"=-5300, "Instrument - Serial Com"=-5301, "Instrument - Camera"=-5302, "Instrument - PS"=-5303, "Instrument - Oscilloscope"=-5304, "Instrument - Function Gen"=-5305, "Instrument - Load"=-5306, "Instrument - Meter"=-5307, "Instrument - Power Control"=-5308, "Instrument - Motion"=-5309, "Instrument - RF"=-5310, "System Exe"=-5400, "Image Processing"=-5500, "Communication"=-5600, "Script - Syntax Error"=-6000, "Script - Invalid Name or Param"=-6100, "Script - Timeout"=-6200, "Invalid Data"=-6300] ("Std Code")
                        n2160 = Format Into String(format string="Warning, Remote Test request attempted to set to nonexistant sequence: \"%s\"." ("Description"), w4571) -> (resulting string=w4572:string)  [unwired: 2 in, 1 out]
                        n2161 = call "Error.Set-Change Error Info.vi"("Std Code"=w4574, "Description"=w4572, "Set Error"=TRUE) -> ("error out"=w4570:errorcluster)  [unwired: 8 in]
                      }
                      frame 0, Default {
                        n2162 = To Unsigned Word Integer(number=w4577) -> (unsigned 16bit integer=w4578:u16)
                        n2163 = property on="Sequence" class="Ring (strict)"("Value"=w4578) -> ()  [unwired: 2 in, 2 out]
                      }
                    }
                  }
                }
                n2164 = case shown="No Error" w4556 {
                  selector: w4556 -> [_ w4596]
                  tunnel: w4561 -> [w4590 w4595]
                  tunnel: w4558 -> [w4589 _]
                  tunnel: w4560 -> [w4588 w4599]
                  tunnel: [w4587 w4599] -> w4559
                  tunnel: w4555 -> [w4581 _]
                  tunnel: w4554 -> [w4580 _]
                  frame No Error {
                    (unwired) TRUE ("Log")
                    n2165 = Unbundle By Name(w4589) -> ("SN"=w4579:string, "Pos"=w4586:string)
                    n2166 = local write "Position"(w4586) -> ()
                    n2167 = local write "SN"(w4579) -> ()
                    n2168 = local write "SN Rslt"(w4579) -> ()
                    n2169 = Empty String/Path?(string/path=w4586) -> (empty?=w4585:bool)
                    n2170 = Format Into String(format string="Remote Test Launch: Seq = %s, SN = %s" ("Message"), w4580, w4579) -> (resulting string=w4583:string)  [unwired: 2 in, 1 out]
                    n2171 = call <vilib>:"Q.Enqueue Seq.vi"("Seq Task Name"="Test Reset" ("Task Name"), "Q In"=w4590) -> ("Q Out"=w4591:refnum<queue>)  [unwired: 8 in, 1 out]
                    n2172 = Unbundle By Name(w4581) -> ("Log"=w4584:refnum<class "Event Notification.lvclass">)
                    n2173 = Bundle By Name(cluster=w4588, "RptUUT.UUTInfo.SN"=w4579, "RptUUT.Position"=w4586) -> (w4587:T73)
                    n2174 = case shown="False" w4585 {
                      frame False {
                        n2175 = property on="Position" class="Str"("Visible"=TRUE) -> ()  [unwired: 2 in, 2 out]
                      }
                      frame True {
                      }
                    }
                    n2176 = call <vilib>:"Q.Enqueue Seq.vi"("Seq Task Name"="Test Start", "Q In"=w4591) -> ()  [unwired: 8 in, 2 out]
                    n2177 = call <vilib>:"Event Notification.Status Message.vi"("Message"=w4583, "Event Notification in"=w4584) -> ()  [unwired: 10 in]
                  }
                  frame Error {
                    n2178 = Bundle By Name(cluster=w4596, "status"=FALSE) -> (w4598:errorcluster)
                    n2179 = call "TestExec.Health, Set Warning.vi"("Error"=w4598, "Q In"=w4595) -> ()  [unwired: 9 in, 1 out]
                  }
                }
              }
            }
          }
          frame "Test Start" {
            n2180 = property on="Sequence" class="Ring (strict)"() -> ("RingText.Text"=w4650:string)  [unwired: 2 in, 2 out]
            n2181 = local read "SN"() -> (w4632:string)
            n2182 = local write "Funct Tab"(0) -> ()
            n2183 = Unbundle By Name(w4604) -> ("Cfg.Dirs.Logs"=w4606:path)
            n2184 = Unbundle By Name(w4603) -> ("Opts.SetOpts"=w4613:bool)
            n2185 = To Variant(anything=TRUE) -> (Variant=w4655:variant)
            n2186 = Unbundle By Name(w4604) -> ("Log"=w4624:refnum<class "Event Notification.lvclass">)
            n2187 = Format Into String(format string="*** Starting Test Sequence %s, SN: %s" ("Message"), w4650, w4632) -> (resulting string=w4623:string)  [unwired: 2 in, 1 out]
            n2188 = call <vilib>:"Q.Enqueue App.vi"("Data1"=w4655, "Task Name"="Lock Test Controls", "Q In"=w4651) -> ("Q Out"=w4612:refnum<queue>)  [unwired: 7 in, 1 out]
            n2189 = call "TestExec.Event Counter Log.vi"("Root Name"="Test Cycle Count", "Log Folder"=w4606) -> ("Event Cnt Out"=w4607:i32)  [unwired: 9 in]
            n2190 = case shown="False" w4613 {
              frame False {
                n2191 = local write "Funct Tab"(0) -> ()
              }
              frame True {
              }
            }
            n2192 = local write "Total Test Cycles"(w4607) -> ()
            n2193 = call <vilib>:"Q.Enqueue Seq.vi"("Seq Task Name"="Init Params" ("Task Name"), "Q In"=w4612) -> ("Q Out"=w4611:refnum<queue>)  [unwired: 8 in, 1 out]
            n2194 = call <vilib>:"Event Notification.Status Message.vi"("Log"=TRUE, "Message"=w4623, "Event Notification in"=w4624) -> ()  [unwired: 9 in]
            n2195 = call <vilib>:"Q.Enqueue Task.vi"("Task Name"="StaTest Start", "Q In"=w4611) -> ("Q Out"=w4610:refnum<queue>)  [unwired: 8 in, 1 out]
            n2196 = Unbundle By Name(w4603) -> ("SeqMgr"=w4646:refnum<class "SeqMgr.lvclass">, "Sequences"=w4648:T66[])
            n2197 = Unbundle By Name(w4603) -> ("CfgFilePaths.ScriptLibDirs"=w4602:path[])
            n2198 = To Long Integer(number="Sequence") -> (32bit integer=w4639:i32)
            n2199 = call <vilib>:"Q.Enqueue Task.vi"("Task Name"="Sta Test Mode", "Q In"=w4610) -> ("Q Out"=w4618:refnum<queue>)  [unwired: 8 in, 1 out]
            n2200 = invoke on="Abort Flag" class="Bool (strict)" method="Reinit To Default"() -> ()  [unwired: 3 in, 3 out]
            n2201 = Index Array(array=w4648, index=w4639) -> (element=w4647:T66)
            n2202 = call <vilib>:"Q.Enqueue Task.vi"("Task Name"="Sta Notify", "Q In"=w4618) -> ("Q Out"=w4614:refnum<queue>)  [unwired: 8 in, 1 out]
            n2203 = Unbundle By Name(w4647) -> ("Name"=w4627:string, "Path"=w4619:path)
            "Seq Rslt" <- w4627
            n2204 = Strip Path(path=w4619) -> (stripped path=w4620:path)  [unwired: 1 out]
            n2205 = Bundle By Name(cluster=w4603, "CfgFilePaths.CurSeqDir"=w4620) -> (w4621:T73)
            n2206 = call <vilib>:"Q.Enqueue Seq.vi"("Seq Task Name"="Test Running" ("Task Name"), "Q In"=w4614) -> ()  [unwired: 8 in, 2 out]
            n2207 = local write "Test State"(enum32{"Idle", "Running", "Completed"}."Running" ("Test State")) -> ()
            n2208 = property on="Pause" class="Bool (strict)"() -> ("Value"=w4633:bool)  [unwired: 2 in, 2 out]
            n2209 = call <vilib>:"SeqMgr.Sequence Load.vi"("Seq Source Search Folders"=w4602, "File Path"=w4619) -> ("error out"=w4637:errorcluster, "PN"=→"SeqPN":string, "Name"=→"SeqName":string, "Seq Steps"=w4626:string[][], "Ver"=→"SeqVer":string)  [unwired: 5 in]
            "Script" <- w4626
            n2210 = call <vilib>:"SeqMgr.Start Sequence.vi"("SeqSteps"=w4626, "Name"=w4627, "SeqMgr in"=w4646) -> ("Start Time"=w4638:timestamp, "SeqMgr out"=w4656:refnum<class "SeqMgr.lvclass">)  [unwired: 5 in, 2 out]
            n2211 = case shown="True" w4633 {
              frame False {
              }
              frame True {
                n2212 = property on="Inc Step" class="Bool"("DisabledEnum"=T36."Enabled" ("Disabled")) -> ()  [unwired: 2 in, 2 out]
                n2213 = property on="Step Run" class="Bool"("DisabledEnum"=T36."Enabled" ("Disabled")) -> ()  [unwired: 2 in, 2 out]
              }
            }
            n2214 = property on="Mode" class="Ring (strict)"() -> ("RingText.Text"=w4631:string)  [unwired: 2 in, 2 out]
            n2215 = Bundle By Name(cluster=w4621, "ResultState"=T63 {"State"=enum."Passing", "Code"=0, "Description"=""} ("Result Info"), "SeqMgr"=w4656) -> (w4645:T73)
            n2216 = local read "PN"() -> (w4608:string)
            n2217 = local read "SN"() -> (w4615:string)
            "SN Rslt" <- w4615
            n2218 = local read "Operator"() -> (w4630:string)
            n2219 = local write "PLC Running"(FALSE ("PLC Running")) -> ()
            n2220 = Bundle By Name(cluster=w4645, "RptHdr.Test Run.Start Time"=w4638, "RptHdr.Test Sequence.Name"=w4627, "ResultError"=w4637, "RptHdr.Test Sequence.Config"=T62 {"Config_Item"=[]} ("RptHdrInfo.Test Sequence.Config"), "RptHdr.Test Run.Operator"=w4630, "RptHdr.Test Run.Mode"=w4631, "RptUUT.UUTInfo.SN"=w4615, "RptUUT.UUTInfo.PN"=w4608, "Repeat(s)"=-1.0, "Lists.CmtPrmpt"=FALSE) -> (w4644:T73)
            n2221 = invoke on="Results Table" class="Arr (strict)" method="Reinit To Default"() -> ()  [unwired: 3 in, 3 out]
            n2222 = invoke on="Progress 2" class="Slide (strict)" method="Reinit To Default"() -> ()  [unwired: 3 in, 3 out]
          }
          frame "Init Params" {
            w4723 = u32 13816530
            w4724 = T36."Disabled" ("Disabled")
            w4709 = TRUE ("Top of Q")
            # "TODO - Lookup Process Step based on Sequence"
            # "Empty Data File Folder"
            n2223 = Unbundle By Name(w4689) -> ("SeqMgr"=w4734:refnum<class "SeqMgr.lvclass">, "Opts.ContOnFail"=w4708:bool, "Opts.ContOnErr"=w4707:bool)
            n2224 = Unbundle By Name(w4689) -> ("CfgFilePaths.CurSeqDir"=w4688:path)
            n2225 = Unbundle By Name(w4690) -> ("Cfg.Dirs.Reports"=w4720:path)
            n2226 = Unbundle By Name(w4690) -> ("Cfg.Dirs.Config"=w4687:path)
            n2227 = local read "SeqName"() -> (w4704:string)
            n2228 = local read "SeqVer"() -> (w4702:string)
            n2229 = local read "SeqPN"() -> (w4703:string)
            n2230 = call <vilib>:"Q.Enqueue Task.vi"("Top of Q"=w4709, "Task Name"="Read Limits", "Q In"=w4695) -> ("Q Out"=w4726:refnum<queue>)  [unwired: 7 in, 1 out]
            n2231 = Not(x=w4708) -> (.not. x?=w4706:bool)
            n2232 = Not(x=w4707) -> (.not. x?=w4705:bool)
            n2233 = Bundle By Name(cluster=T31 {"Name"="", "PN"="", "Version"="", "Note"=""} ("Software Items"), "Name"=w4704, "PN"=w4703, "Version"=w4702) -> (w4712:T31)
            n2234 = call <vilib>:"Q.Enqueue Task.vi"("Top of Q"=w4709, "Task Name"="Sta Set TimeOut", "Q In"=w4726) -> ("Q Out"=w4700:refnum<queue>)  [unwired: 7 in, 1 out]
            n2235 = Build Path(base path=w4720, name or relative path="Current Test Data Files") -> (appended path=w4698:path)
            n2236 = Path To String(path=w4688) -> (string=w4685:string)
            n2237 = Path To String(path=w4687) -> (string=w4686:string)
